vi "0~20mA Conv.vi"(1 "Register Value":u16) -> (0 "Current mA":dbl)   [LabVIEW 2024]
doc: "Convert analogue register value to 0~20mA value."
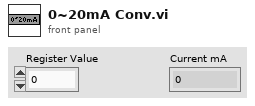
[diagram p1: front panel]
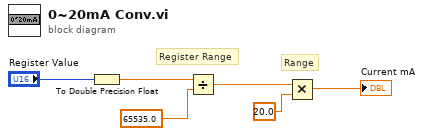
[diagram p0: block diagram]
diagram:
  # "Register Range"
  # "Range"
  n1 = To Double Precision Float(number="Register Value") -> (double precision float=w2:dbl)
  n2 = Divide(x=w2, y=65535.0) -> (x/y=w5:dbl)
  n3 = Multiply(x=w5, y=20.0) -> (x*y=→"Current mA":dbl)
